vi "SendSWtrigger_5782.vi"(8 "error in":errorcluster, 11 "scope in":T1) -> (0 "error out":errorcluster, 3 "scope out":T1)   [LabVIEW 2013]
uses:
  controls/scope_params_5782.ctl
  Utilities/Ticker/Ticker.lvclass
  Scope/controls/ScopeMode.ctl
  Config/FPGAref_5782.ctl
  FPGA/DataMode.ctl
  controls/5782_trigger_type.ctl
  <vilib>/rvi/interface/common/niFpgaWaitOnOcc.vi
  <vilib>/Utility/error.llb/Error Cluster From Error Code.vi
  <vilib>/rvi/errors/niLvFpgaAdjustHostInterfaceError.vi
  <vilib>/rvi/interface/nirviReadWriteControl/nirviReadWriteControl.xnode
  NiFpgaLv.dll
  <vilib>/rvi/interface/Simulation/niFpgaSimulationCallBeginRW.vi
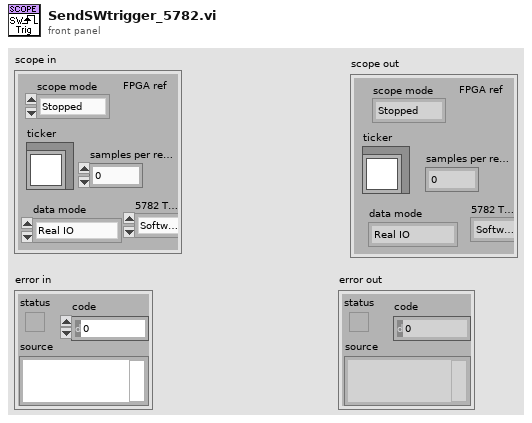
[diagram p1: front panel]
types:
  T1 = typedef "scope_params_5782.ctl" = cluster{"scope mode":T2, "ticker":refnum<class "Ticker.lvclass">, "samples per record":i32, "FPGA ref":T3, "data mode":T4, "5782 Trigger":T5}
  T2 = typedef "ScopeMode.ctl" = enum16{"Stopped", "Single", "Running"}
  T3 = typedef "FPGAref_5782.ctl" = refnum<k20>
  T4 = typedef "DataMode.ctl" = enum16{"Real IO", "Simulated"}
  T5 = typedef "5782_trigger_type.ctl" = enum16{"Software", "Trigger input"}
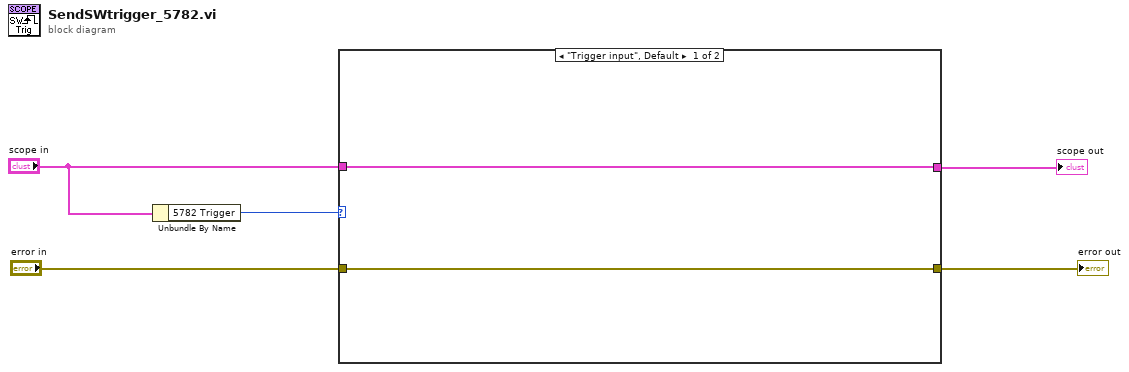
[diagram p0: block diagram]
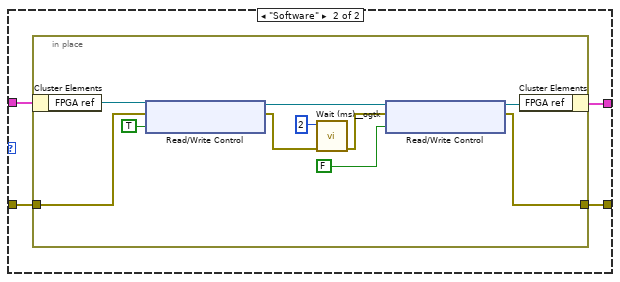
[diagram p2: hidden frame]
diagram:
  n1 = Unbundle By Name("scope in") -> ("5782 Trigger"=w5:T5)
  n2 = case shown="\"Trigger input\", Default" w5 {
    tunnel: "scope in" -> [w7 w11]
    tunnel: [w7 w10] -> w3
    tunnel: "error in" -> [w6 w9]
    tunnel: [w6 w8] -> w1
    frame "Trigger input", Default {
    }
    frame "Software" {
      n3 = in-place {
        in-place-border: w9 -> [w19]
        in-place-border: [w12] -> w8
        n4 = in-place-cluster #1(w11) -> ("FPGA ref"=w21:T3)
        n5 = xnode "Read/Write Control"("FPGA VI Reference In"=w21, "error in"=w19, "Trigger Acquisition"=TRUE) -> ("FPGA VI Reference Out"=w13:T3, "error out"=w18:errorcluster)
        n6 = call <userlib>:"Wait (ms)__ogtk.vi"("error in (no error)"=w18, "milliseconds to wait"=u32 2) -> ("error out"=w16:errorcluster)  [unwired: 8 in, 1 out]
        n7 = xnode "Read/Write Control"("FPGA VI Reference In"=w13, "error in"=w16, "Trigger Acquisition"=FALSE) -> ("FPGA VI Reference Out"=w14:T3, "error out"=w12:errorcluster)
        n8 = in-place-cluster #1("FPGA ref"=w14) -> (w10:T1)
      }
    }
  }
  "scope out" <- w3
  "error out" <- w1
